vi "GetZerothTabableControl.vi"(11 "Controls[]":refnum<vi>[](array[refnum])) -> (3 "Control out":refnum<vi>)   [LabVIEW 2016]
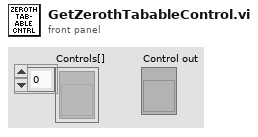
[diagram p1: front panel]
types:
  T1 = enum8{"Enabled", "Disabled", "Disabled and Grayed Out"}
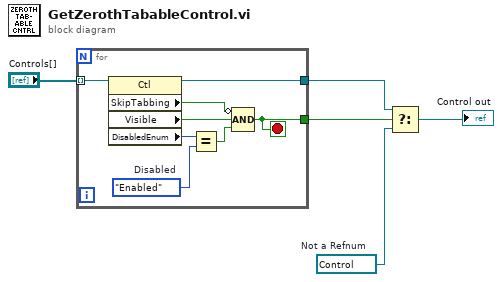
[diagram p0: block diagram]
diagram:
  w1 = refnum<vi> refnum  # Not a Refnum
  n1 = for {
    tunnel: "Controls[]" -> [w7] mode=indexing
    tunnel: [w6] -> w3
    tunnel: [w8] -> w4
    stop <- w8 stop-if-true
    w12 = T1."Enabled"  # Disabled
    n2 = property class="Ctl"(reference=w7) -> (reference out=w6:refnum<vi>, "SkipTabbing"=w11:bool, "Visible"=w9:bool, "DisabledEnum"=w13:T1)  [unwired: 1 in, 1 out]
    n3 = Equal?(x=w13, y=w12) -> (x = y?=w10:bool)
    n4 = Compound Arithmetic op=AND(invert w11, w9, w10) -> (w8:bool)
  }
  n5 = Select(t=w3, s=w4, f=w1) -> (s? t:f=→"Control out":refnum<vi>)
